vi "Perpetual Motion Machine.vi"() -> ()   [LabVIEW 2015]
uses:
  <userlib>/Newport ESP301/Newport ESP301.lvlib
panel:
  in  "?":bool
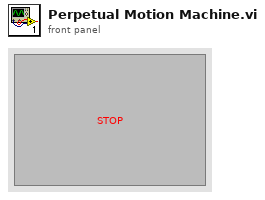
[diagram p1: front panel]
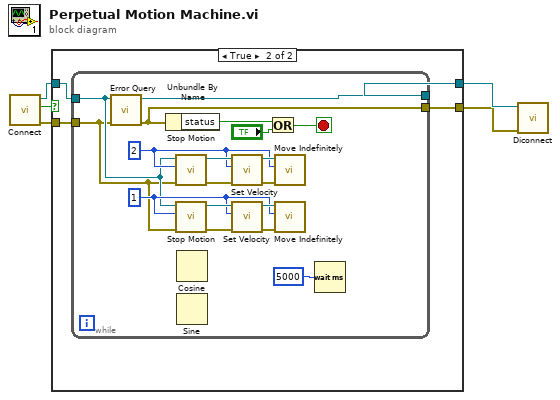
[diagram p0: block diagram]
diagram:
  n1 = call "Connect.vi"() -> ("error out"=w3:errorcluster, "Connected"=w5:bool, "VISA resource name out"=w4:refnum<visa-resource-name>)  [unwired: 5 in]
  n2 = case shown="True" w5 {
    tunnel: w4 -> [w7 w11]
    tunnel: w3 -> [w6 w10]
    tunnel: [w7 w9] -> w2
    tunnel: [w6 w8] -> w1
    frame False {
    }
    frame True {
      n3 = while {
        tunnel: w11 -> [w19]
        tunnel: w10 -> [w18]
        tunnel: [w17] -> w9
        tunnel: [w16] -> w8
        stop <- w13 stop-if-true
        w20 = 2
        w23 = 1
        n4 = call <userlib>:"Error Query.vi"("error in (no error)"=w18, "VISA resource name"=w19) -> ("error out"=w16:errorcluster, "VISA resource name out"=w17:refnum<visa-resource-name>)  [unwired: 2 in, 2 out]
        n5 = Unbundle By Name(w16) -> ("status"=w14:bool)
        n6 = call <userlib>:"Stop Motion.vi"("error in (no error)"=w18, "Axis (1)"=w20, "VISA resource name"=w19) -> ("error out"=w26:errorcluster, "VISA resource name out"=w27:refnum<visa-resource-name>)  [unwired: 3 in]
        n7 = call <userlib>:"Stop Motion.vi"("error in (no error)"=w18, "Axis (1)"=w23, "VISA resource name"=w19) -> ("error out"=w28:errorcluster, "VISA resource name out"=w29:refnum<visa-resource-name>)  [unwired: 3 in]
        n8 = Cosine() -> ()  [unwired: 1 in, 1 out]
        n9 = Sine() -> ()  [unwired: 1 in, 1 out]
        n10 = call <userlib>:"Set Velocity.vi"("error in (no error)"=w26, "Axis (1)"=w20, "VISA resource name"=w27) -> ("error out"=w21:errorcluster, "VISA resource name out"=w22:refnum<visa-resource-name>)  [unwired: 3 in]
        n11 = call <userlib>:"Set Velocity.vi"("error in (no error)"=w28, "Axis (1)"=w23, "VISA resource name"=w29) -> ("error out"=w24:errorcluster, "VISA resource name out"=w25:refnum<visa-resource-name>)  [unwired: 3 in]
        n12 = Or(x=w14, y="?") -> (x .or. y?=w13:bool)
        n13 = call <userlib>:"Move Indefinitely.vi"("error in (no error)"=w21, "Axis (1)"=w20, "VISA resource name"=w22) -> ()  [unwired: 3 in, 2 out]
        n14 = call <userlib>:"Move Indefinitely.vi"("error in (no error)"=w24, "Axis (1)"=w23, "VISA resource name"=w25) -> ()  [unwired: 3 in, 2 out]
        n15 = Wait (ms)(milliseconds to wait=5000) -> ()  [unwired: 1 out]
      }
    }
  }
  n16 = call "Diconnect.vi"("error in (no error)"=w1, "VISA resource name"=w2) -> ()  [unwired: 6 in]
